vi "Teleop.vi"(10 "Match Info":T2={"Autonomous Elapsed Seconds"=0.0, "TeleOp Elapsed Seconds"=0.0, "Disabled Elapsed Seconds"=0.0, "Visited Autonomous"=FALSE, "Visited TeleOp"=FALSE, "Visited Disabled"=FALSE, "Autonomous Settings"={"Autonomous Style"=enum."Independent", "VI Refnum"=refnum}}, 11 "Call Context":T3) -> ()   [LabVIEW 2019]
doc: "This VI is called for each TeleOp packet received from the DS where the robot is not disabled. It is often used to read from the joysticks and update I/O or to update setpoints for timed control loops. It should complete and return within 20 milliseconds or it may miss DS packets."
uses:
  <vilib>/Rock Robotics/WPI/DriverStation/WPI_DriverStationDerivedRobotMode.ctl
  <vilib>/Rock Robotics/WPI/DriverStation/WPI_DriverStationMatch Info.ctl
  <vilib>/Rock Robotics/SystemInterfaces/DIO/FPGA_DIOPWMChannel.ctl
  <vilib>/Rock Robotics/WPI/Utilities/WPI_GetSetVariantRefNum.vi
  <vilib>/Rock Robotics/WPI/MotorControl/WPI_MotorControlOpen VictorSP.vi
  <vilib>/Rock Robotics/Network Tables/NT Write Numeric Array.vi
  <vilib>/Rock Robotics/Network Tables/NT Read Boolean.vi
  <vilib>/Rock Robotics/Network Tables/NT Read Number.vi
  <vilib>/Rock Robotics/Network Tables/NT Write Boolean Array.vi
panel:
  in  "45 % DC":bool
  in  "35 % DC":bool
  in  "25 % DC":bool
  in  "PWM Channel":T1
  out "Sample Slider 0":dbl(slide) scale=0.0..5.0
  out "Sample Boolean 1":bool
  out "Sample Boolean 0":bool
  # "(Duty cycle basically means how fast the motor is spinning)"
  # "Use the PWM Channel control to change which PWM slot is in use on the RoboRIO."
  # "If the 45 % button is pressed AND Button 1 (X) is pressed, rotate motor at 45 % duty cycle."
  # "If the 25 % button is pressed AND Button 1 (X) is pressed, rotate motor at 25 % duty cycle."
  # "If the 35 % button is pressed AND Button 1 (X) is pressed, rotate motor at 35 % duty cycle."
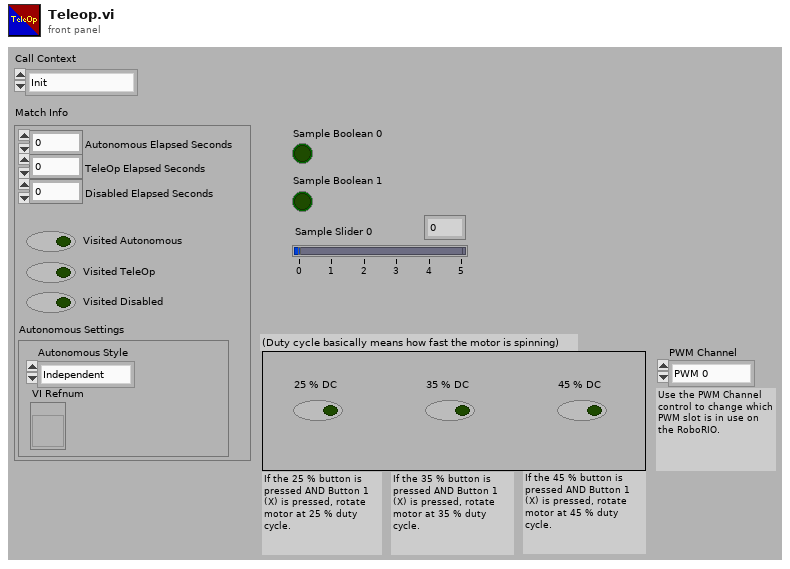
[diagram p1: front panel]
types:
  T1 = typedef "FPGA_DIOPWMChannel.ctl" = enum8{"PWM 0", "PWM 1", "PWM 2", "PWM 3", "PWM 4", "PWM 5", "PWM 6", "PWM 7", "PWM 8", "PWM 9", "PWM MXP 0", "PWM MXP 1", "PWM MXP 2", "PWM MXP 3", "PWM MXP 4", "PWM MXP 5", "PWM MXP 6", "PWM MXP 7", "PWM MXP 8", "PWM MXP 9", "Invalid"}
  T2 = typedef "WPI_DriverStationMatch Info.ctl" = cluster{"Autonomous Elapsed Seconds":dbl, "TeleOp Elapsed Seconds":dbl, "Disabled Elapsed Seconds":dbl, "Visited Autonomous":bool, "Visited TeleOp":bool, "Visited Disabled":bool, "Autonomous Settings":cluster{"Autonomous Style":enum16{"Iterative", "Independent"}, "VI Refnum":refnum<vi>}}
  T3 = typedef "WPI_DriverStationDerivedRobotMode.ctl" = enum16{"Init", "Execute", "Stop"}
  T4 = typedef "WPI_JoystickDevRef.ctl" = cluster{"Device":T5}
  T5 = typedef "WPI_JoystickDeviceEnum.ctl" = enum16{"USB 0", "USB 1", "USB 2", "USB 3", "USB 4", "USB 5"}
  T6 = typedef "WPI_RobotDriveDevRef.ctl" = cluster{"DevStatus":errorcluster, "Motors[]":T7[], "Square Inputs":bool, "Max Output":dbl}
  T7 = typedef "WPI_MotorControlDeviceRef.ctl" = cluster{"DeviceStatus":errorcluster, "Type":T8, "PWM":cluster{"PWM Channel":T1, "DeadBand":T9}, "CAN":cluster{"Device Number":u8, "SetOutput VI Ref":variant, "GetOutput VI Ref":variant, "Enable VI Ref":variant, "Disable VI Ref":variant, "Data":variant}, "Invert":bool, "DIO PWM":cluster{"PWM \"Enable\" Channel":T1, "DIOChannel":T10, "PWM Rate":dbl}}
  T8 = typedef "WPI_MotorControlType.ctl" = enum16{"PWM", "CAN", "DIO PWM"}
  T9 = typedef "WPI_PWMDeadband.ctl" = cluster{"Name":string, "maxPositivePwm":i32, "minPositivePwm":i32, "centerPwm":i32, "maxNegativePwm":i32, "minNegativePwm":i32, "angularRange":u16}
  T10 = typedef "FPGA_DIOChannel.ctl" = enum8{"DIO 0", "DIO 1", "DIO 2", "DIO 3", "DIO 4", "DIO 5", "DIO 6", "DIO 7", "DIO 8", "DIO 9", "DIO MXP 0", "DIO MXP 1", "DIO MXP 2", "DIO MXP 3", "DIO MXP 4", "DIO MXP 5", "DIO MXP 6", "DIO MXP 7", "DIO MXP 8", "DIO MXP 9", "DIO MXP 10", "DIO MXP 11", "DIO MXP 12", "DIO MXP 13", "DIO MXP 14", "DIO MXP 15", "SPI Port CS1", "SPI Port CS2", "SPI Port CS3", "SPI Port MISO", "SPI Port MOSI", "Invalid"}
  T11 = cluster{"JoystickDevRef":T4, "RobotDriveDevRef":T6}
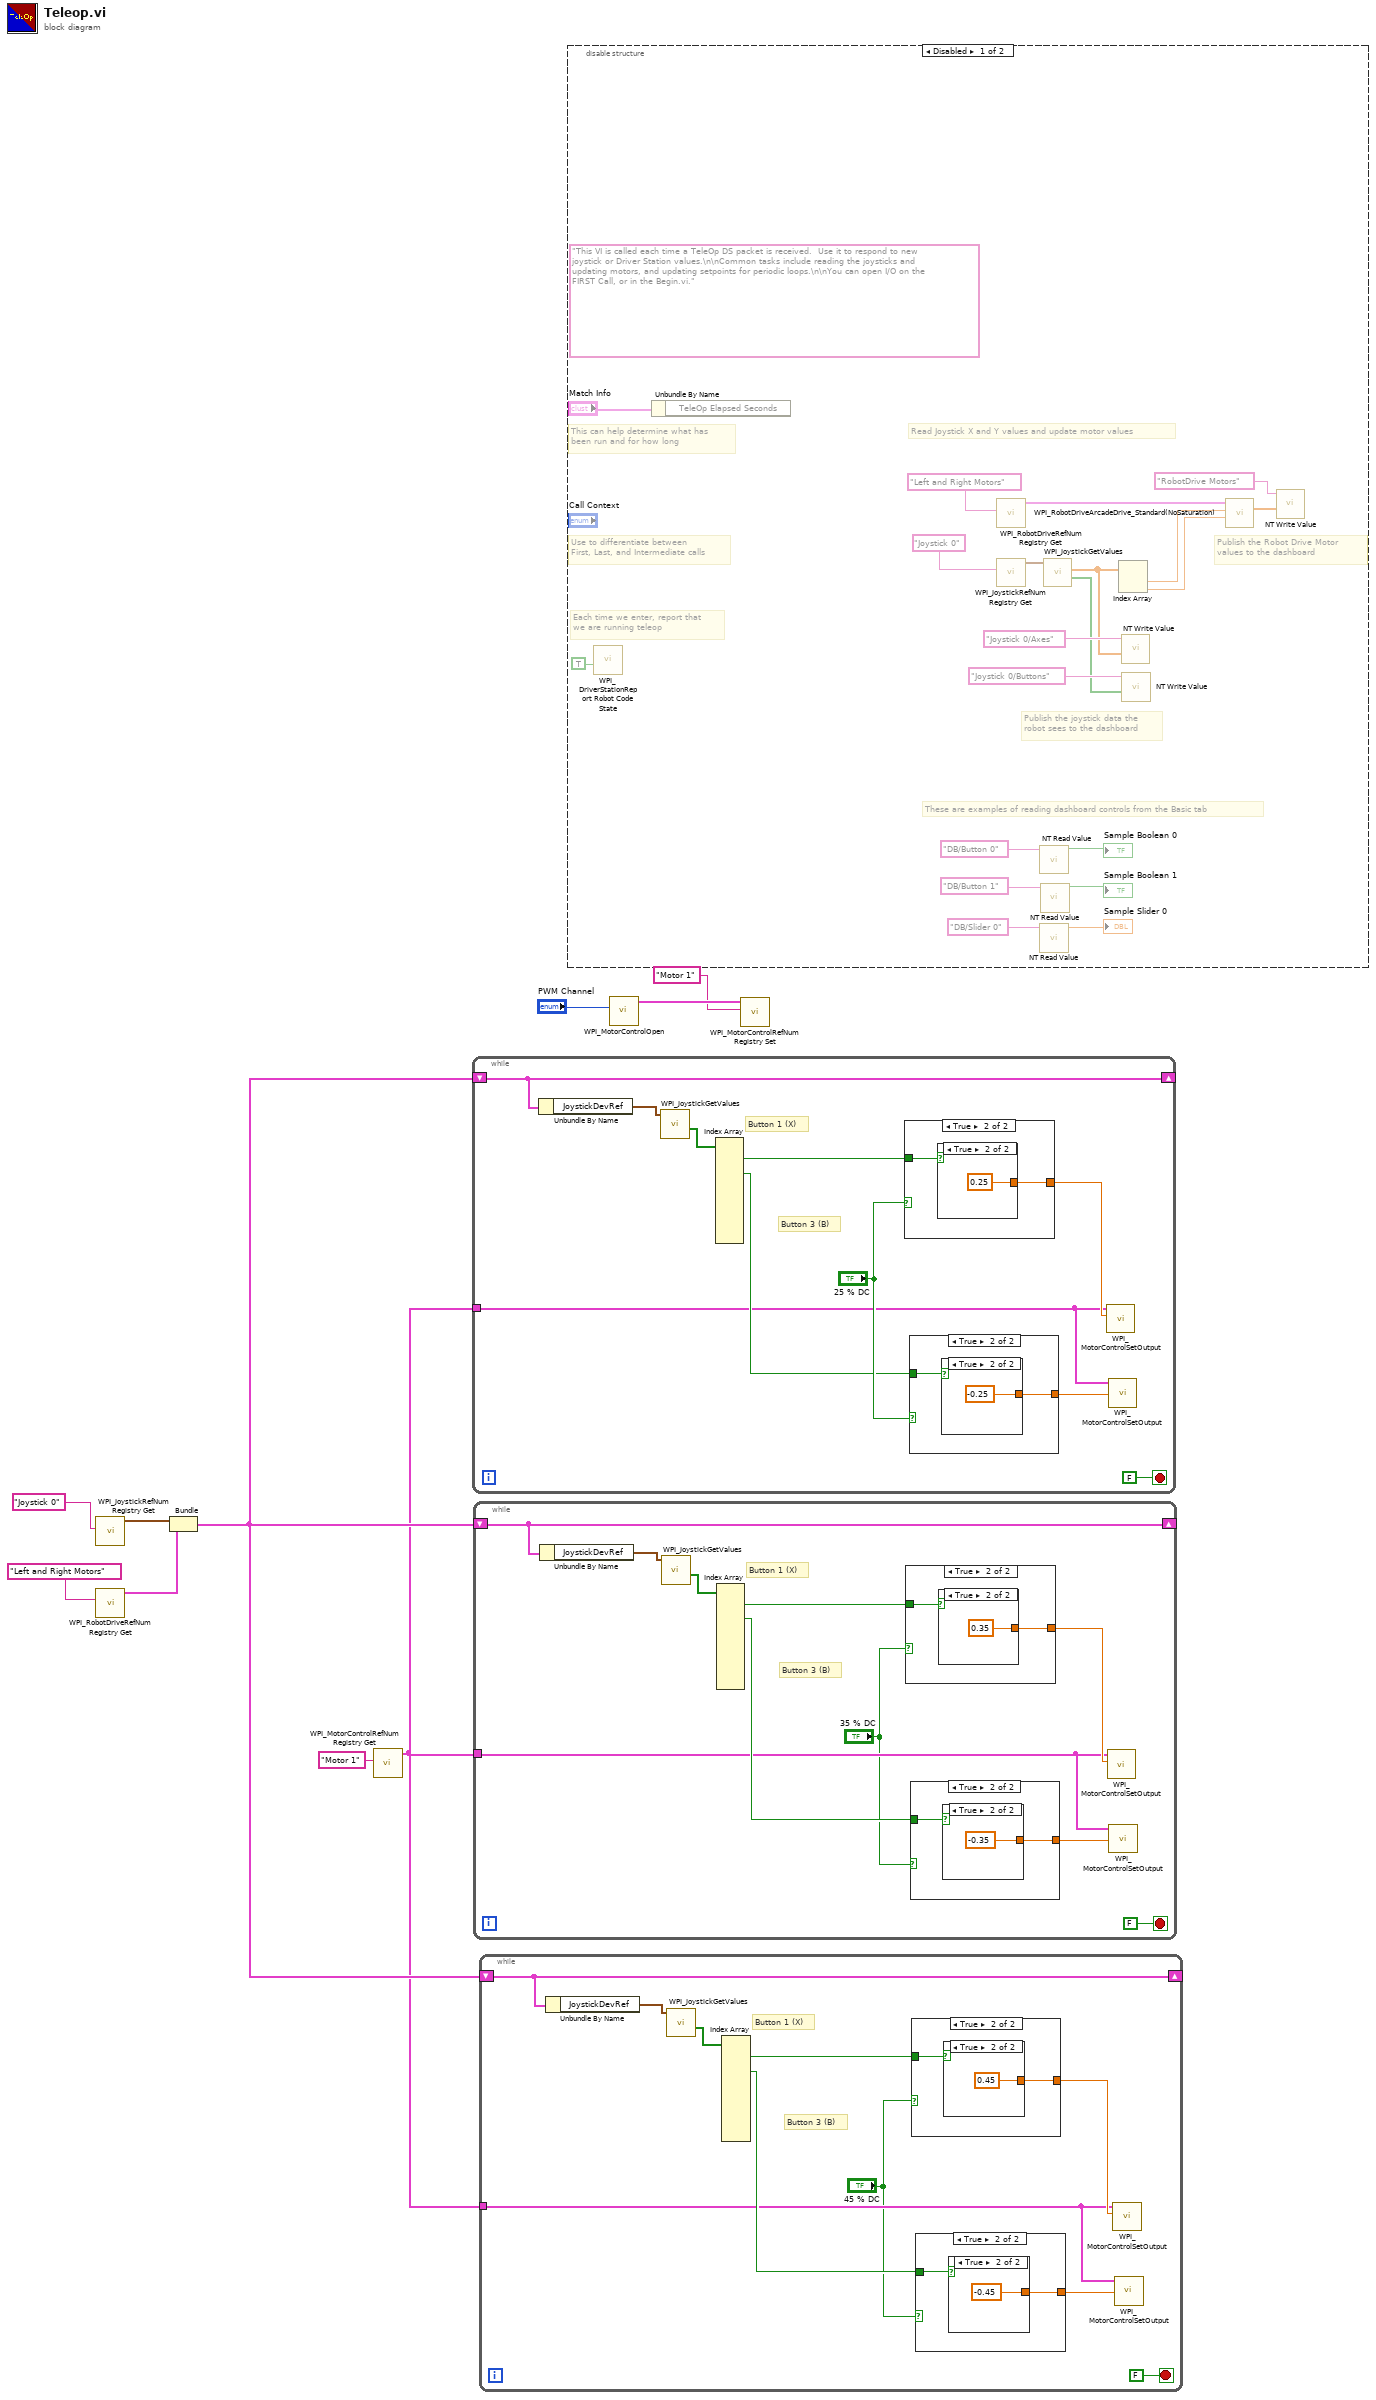
[diagram p0: block diagram]
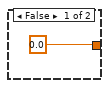
[diagram p2: hidden frame]
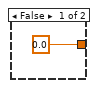
[diagram p3: hidden frame]
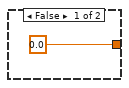
[diagram p4: hidden frame]
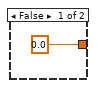
[diagram p5: hidden frame]
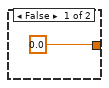
[diagram p6: hidden frame]
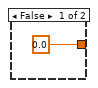
[diagram p7: hidden frame]
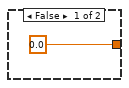
[diagram p8: hidden frame]
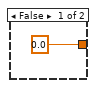
[diagram p9: hidden frame]
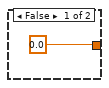
[diagram p10: hidden frame]
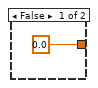
[diagram p11: hidden frame]
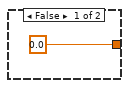
[diagram p12: hidden frame]
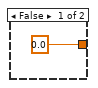
[diagram p13: hidden frame]
diagram:
  n1 = call <vilib>:"WPI_JoystickRefNum Registry Get.vi"("refnum name"="Joystick 0") -> ("JoystickDevRef"=w9:T4)  [unwired: 1 in, 9 out]
  n2 = call <vilib>:"WPI_RobotDriveRefNum Registry Get.vi"("refnum name"="Left and Right Motors") -> ("RobotDriveDevRef"=w8:T6)  [unwired: 1 in, 9 out]
  n3 = Bundle("JoystickDevRef"=w9, "RobotDriveDevRef"=w8) -> (w2:T11)  [unwired: 1 out]
  n4 = call <vilib>:"WPI_MotorControlRefNum Registry Get.vi"("refnum name"="Motor 1") -> ("MotorControlDevRef"=w1:T7)  [unwired: 9 in, 1 out]
  n5 = while {
    tunnel: w1 -> [w13]
    shift-right: [w20] -> _
    shift-left: w2 -> [w20]
    stop <- FALSE stop-if-true
    # "Button 3 (B)"
    # "Button 1 (X)"
    n6 = Unbundle By Name(w20) -> ("JoystickDevRef"=w19:T4)
    n7 = call <vilib>:"WPI_JoystickGetValues.vi"("JoystickDevRef"=w19) -> ("Buttons"=w18:bool[])  [unwired: 6 in, 4 out]
    n8 = Index Array(array=w18) -> (element #1=w17:bool, element #3=w14:bool)  [unwired: 12 in, 10 out]
    n9 = case shown="True" "25 % DC" {
      tunnel: w17 -> [_ w28]
      tunnel: [0.0 ("Output") w27] -> w16
      frame False {
      }
      frame True {
        n10 = case shown="True" w28 {
          tunnel: [0.0 ("Output") 0.25 ("Output")] -> w27
          frame False {
          }
          frame True {
          }
        }
      }
    }
    n11 = case shown="True" "25 % DC" {
      tunnel: w14 -> [_ w23]
      tunnel: [0.0 ("Output") w22] -> w12
      frame False {
      }
      frame True {
        n12 = case shown="True" w23 {
          tunnel: [0.0 ("Output") -0.25 ("Output")] -> w22
          frame False {
          }
          frame True {
          }
        }
      }
    }
    n13 = call <vilib>:"WPI_MotorControlSetOutput.vi"("Output"=w16, "MotorControlDevRef"=w13) -> ()  [unwired: 7 in, 3 out]
    n14 = call <vilib>:"WPI_MotorControlSetOutput.vi"("Output"=w12, "MotorControlDevRef"=w13) -> ()  [unwired: 7 in, 3 out]
  }
  n15 = while {
    tunnel: w1 -> [w34]
    shift-right: [w40] -> _
    shift-left: w2 -> [w40]
    stop <- FALSE stop-if-true
    # "Button 3 (B)"
    # "Button 1 (X)"
    n16 = Unbundle By Name(w40) -> ("JoystickDevRef"=w39:T4)
    n17 = call <vilib>:"WPI_JoystickGetValues.vi"("JoystickDevRef"=w39) -> ("Buttons"=w38:bool[])  [unwired: 6 in, 4 out]
    n18 = Index Array(array=w38) -> (element #1=w37:bool, element #3=w35:bool)  [unwired: 12 in, 10 out]
    n19 = case shown="True" "35 % DC" {
      tunnel: w37 -> [_ w48]
      tunnel: [0.0 ("Output") w47] -> w36
      frame False {
      }
      frame True {
        n20 = case shown="True" w48 {
          tunnel: [0.0 ("Output") 0.35 ("Output")] -> w47
          frame False {
          }
          frame True {
          }
        }
      }
    }
    n21 = case shown="True" "35 % DC" {
      tunnel: w35 -> [_ w43]
      tunnel: [0.0 ("Output") w42] -> w33
      frame False {
      }
      frame True {
        n22 = case shown="True" w43 {
          tunnel: [0.0 ("Output") -0.35 ("Output")] -> w42
          frame False {
          }
          frame True {
          }
        }
      }
    }
    n23 = call <vilib>:"WPI_MotorControlSetOutput.vi"("Output"=w36, "MotorControlDevRef"=w34) -> ()  [unwired: 7 in, 3 out]
    n24 = call <vilib>:"WPI_MotorControlSetOutput.vi"("Output"=w33, "MotorControlDevRef"=w34) -> ()  [unwired: 7 in, 3 out]
  }
  n25 = while {
    tunnel: w1 -> [w54]
    shift-right: [w60] -> _
    shift-left: w2 -> [w60]
    stop <- FALSE stop-if-true
    # "Button 3 (B)"
    # "Button 1 (X)"
    n26 = Unbundle By Name(w60) -> ("JoystickDevRef"=w59:T4)
    n27 = call <vilib>:"WPI_JoystickGetValues.vi"("JoystickDevRef"=w59) -> ("Buttons"=w58:bool[])  [unwired: 6 in, 4 out]
    n28 = Index Array(array=w58) -> (element #1=w57:bool, element #3=w55:bool)  [unwired: 12 in, 10 out]
    n29 = case shown="True" "45 % DC" {
      tunnel: w57 -> [_ w68]
      tunnel: [0.0 ("Output") w67] -> w56
      frame False {
      }
      frame True {
        n30 = case shown="True" w68 {
          tunnel: [0.0 ("Output") 0.45 ("Output")] -> w67
          frame False {
          }
          frame True {
          }
        }
      }
    }
    n31 = case shown="True" "45 % DC" {
      tunnel: w55 -> [_ w63]
      tunnel: [0.0 ("Output") w62] -> w53
      frame False {
      }
      frame True {
        n32 = case shown="True" w63 {
          tunnel: [0.0 ("Output") -0.45 ("Output")] -> w62
          frame False {
          }
          frame True {
          }
        }
      }
    }
    n33 = call <vilib>:"WPI_MotorControlSetOutput.vi"("Output"=w56, "MotorControlDevRef"=w54) -> ()  [unwired: 7 in, 3 out]
    n34 = call <vilib>:"WPI_MotorControlSetOutput.vi"("Output"=w53, "MotorControlDevRef"=w54) -> ()  [unwired: 7 in, 3 out]
  }
  n35 = disable-structure shown="Disabled" {
    frame Disabled {
      (unwired) "This VI is called each time a TeleOp DS packet is received.  Use it to respond to new joystick or Driver Station values.\n\nCommon tasks include reading the joysticks and updating motors, and updating setpoints for periodic loops.\n\nYou can open I/O on the FIRST Call, or in the Begin.vi."
      # "These are examples of reading dashboard controls from the Basic tab"
      # "Publish the Robot Drive Motor\nvalues to the dashboard"
      # "Publish the joystick data the\nrobot sees to the dashboard"
      # "Each time we enter, report that\nwe are running teleop"
      # "Use to differentiate between\nFirst, Last, and Intermediate calls"
      # "This can help determine what has\nbeen run and for how long"
      # "Read Joystick X and Y values and update motor values"
      n36 = call <vilib>:"WPI_DriverStationReport Robot Code State.vi"("TeleOp"=TRUE ("Autonomous")) -> ()  [unwired: 10 in, 1 out]
      n37 = Unbundle By Name("Match Info") -> ()  [unwired: 1 out]
      n38 = call <vilib>:"WPI_RobotDriveRefNum Registry Get.vi"("refnum name"="Left and Right Motors") -> ("RobotDriveDevRef"=w88:T6)  [unwired: 1 in, 9 out]
      n39 = call <vilib>:"WPI_JoystickRefNum Registry Get.vi"("refnum name"="Joystick 0") -> ("JoystickDevRef"=w85:T4)  [unwired: 1 in, 9 out]
      n40 = call-poly <vilib>:"NT Read Value.vi"("Name"="DB/Button 0" ("refnum name")) -> ("Boolean"=→"Sample Boolean 0":bool)  [unwired: 9 in, 1 out]
      n41 = call-poly <vilib>:"NT Read Value.vi"("Name"="DB/Slider 0" ("refnum name")) -> ("Numeric"=→"Sample Slider 0":dbl)  [unwired: 9 in, 1 out]
      n42 = call-poly <vilib>:"NT Read Value.vi"("Name"="DB/Button 1" ("refnum name")) -> ("Boolean"=→"Sample Boolean 1":bool)  [unwired: 9 in, 1 out]
      n43 = call <vilib>:"WPI_JoystickGetValues.vi"("JoystickDevRef"=w85) -> ("Buttons"=w79:bool[], "Axes"=w80:dbl[])  [unwired: 6 in, 3 out]
      n44 = Index Array(array=w80) -> (element #1=w87:dbl, element #2=w83:dbl)  [unwired: 2 in]
      n45 = call-poly <vilib>:"NT Write Value.vi"("Numeric Array"=w80, "Name"="Joystick 0/Axes") -> ()  [unwired: 9 in, 1 out]
      n46 = call-poly <vilib>:"NT Write Value.vi"("Boolean Array"=w79, "Name"="Joystick 0/Buttons") -> ()  [unwired: 9 in, 1 out]
      n47 = call <vilib>:"WPI_RobotDriveArcadeDrive_Standard(NoSaturation).vi"("Y axis value"=w83, "X axis value"=w87, "RobotDriveDevRef"=w88) -> ("Motor Values"=w72:dbl[])  [unwired: 1 in, 7 out]
      n48 = call-poly <vilib>:"NT Write Value.vi"("Numeric Array"=w72, "Name"="RobotDrive Motors") -> ()  [unwired: 9 in, 1 out]
    }
    frame Enabled {
    }
  }
  n49 = call-poly <vilib>:"WPI_MotorControlOpen.vi"("PWM Channel"="PWM Channel") -> ("MotorControlDeviceRef"=w5:T7)  [unwired: 9 in, 1 out]
  n50 = call <vilib>:"WPI_MotorControlRefNum Registry Set.vi"("refnum name"="Motor 1", "MotorControlDevRef"=w5) -> ()  [unwired: 8 in, 2 out]
